vi "List Waveforms.vi"(8 "error in (no error)":errorcluster, 10 "Retrieve (All)":enum16{"All", "Non-Volatile"}(ring), 11 "VISA resource name":refnum<visa-resource-name>) -> (0 "error out":errorcluster, 2 "Waveform Names":string[](array[string]), 3 "VISA resource name out":refnum<visa-resource-name>)   [LabVIEW 2017, in "Keithley 3390.lvlib"]
doc: "This VI retrieves a list of the arbitrary waveforms currenty loaded on the instrument."
uses:
  Keithley 3390.lvlib
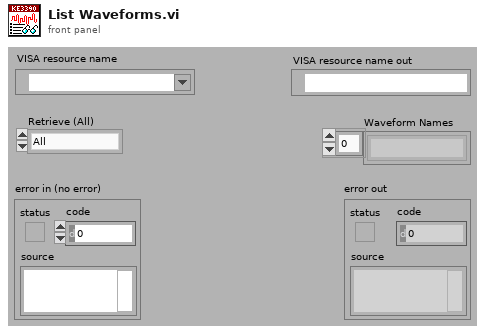
[diagram p1: front panel]
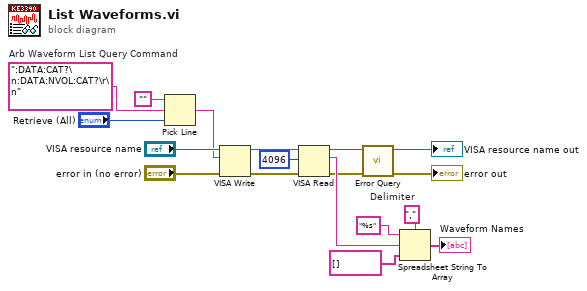
[diagram p0: block diagram]
diagram:
  w6 = ":DATA:CAT?\n:DATA:NVOL:CAT?\r\n"  # Arb Waveform List Query Command
  w12 = ","  # Delimiter
  n1 = Pick Line(string ("")="", multi-line string=w6, line index="Retrieve (All)") -> (output string=w5:string)
  n2 = VISA Write(VISA resource name="VISA resource name", write buffer=w5, error in (no error)="error in (no error)") -> (VISA resource name out=w15:refnum<visa-resource-name>, error out=w14:errorcluster)  [unwired: 1 out]
  n3 = VISA Read(VISA resource name=w15, byte count=u32 4096, error in (no error)=w14) -> (VISA resource name out=w4:refnum<visa-resource-name>, read buffer=w9:string, error out=w1:errorcluster)  [unwired: 1 out]
  n4 = call "Error Query.vi"("error in (no error)"=w1, "VISA resource name"=w4) -> ("error out"=→"error out":errorcluster, "VISA resource name out"=→"VISA resource name out":refnum<visa-resource-name>)  [unwired: 6 in, 2 out]
  n5 = Spreadsheet String To Array(delimiter (Tab)=w12, format string="%s", spreadsheet string=w9, array type (2D Dbl)=string[] []) -> (array=→"Waveform Names":string[])
